vi "ep_Get Significance.vi"(0 "spectra points in window":T4(array[cluster]), 1 "pole pairs":i32, 2 "fundamental frequency [Hz]":dbl, 5 "peaks information":T3(array[cluster]), 7 "enough points for peak search?":bool[](array[boolean]), 9 "number of peaks":i32[](array[numeric]), 11 "error in (no error)":errorcluster, 12 "minimum max-magnitude":dbl, 13 "range of speed":T1) -> (4 "top3 speed data":cluster{"speed [RPM]":dbl, "slip":dbl}[](array[cluster]), 6 "top3 significance":dbl[](array[numeric]), 8 "top3 harmonic for speed calculation":T2[](array[typedef]), 15 "error out":errorcluster)   [LabVIEW 2014, in "NI_EP_Motor Monitoring.lvlib"]
uses:
  <vilib>/addons/Electrical Power/Motor Monitoring/NI_EP_Motor Monitoring.lvlib
  <vilib>/addons/Electrical Power/Motor Monitoring/subVIs/ep_Harmonic for Speed Calculation.ctl
  <vilib>/Analysis/baseanly.llb/Mean (DBL).vi
  <vilib>/Analysis/NI_AALBase.lvlib
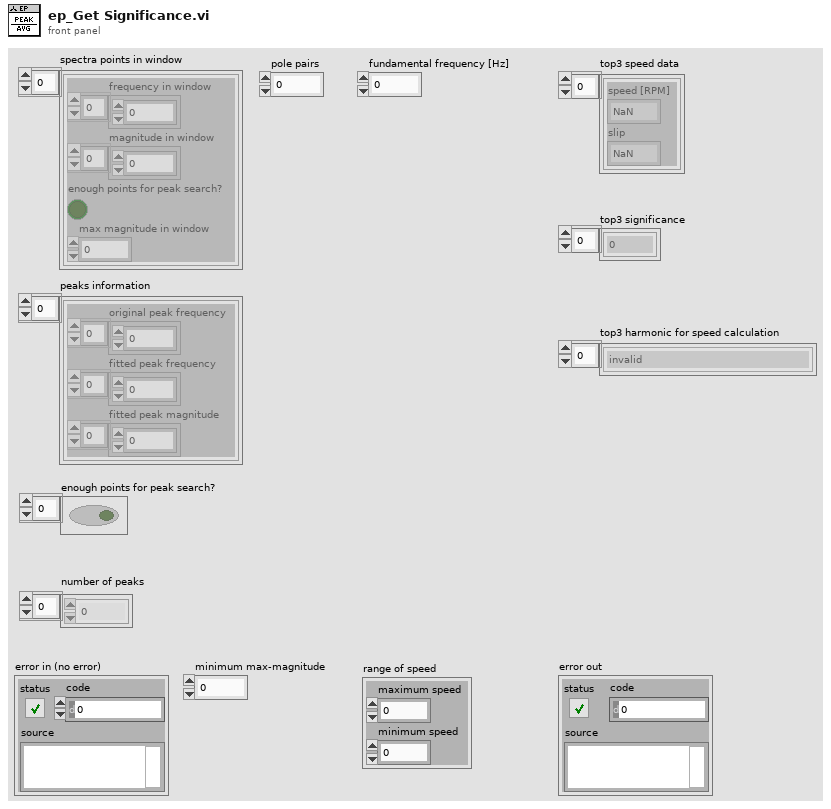
[diagram p1: front panel]
types:
  T1 = cluster{"maximum speed":dbl, "minimum speed":dbl}
  T2 = typedef "NI_EP_Motor Monitoring.lvlib/ep_Harmonic for Speed Calculation.ctl" = enum16{"invalid", "fr", "2fs-2fr", "2fs-fr", "2fr"}
  T3 = cluster{"original peak frequency":dbl[], "fitted peak frequency":dbl[], "fitted peak magnitude":dbl[]}[]
  T4 = cluster{"frequency in window":dbl[], "magnitude in window":dbl[], "enough points for peak search?":bool, "max magnitude in window":dbl}[]
  T5 = typedef "NI_EP_Motor Monitoring.lvlib/ep_Case for Speed Calculation.ctl" = enum16{"no available harmonic for speed calculation", "use the harmonic with highest magnitude", "use the harmonic with highest significance"}
  T6 = cluster{"frequency in window":dbl[], "magnitude in window":dbl[], "enough points for peak search?":bool, "max magnitude in window":dbl}
  T7 = cluster{"maximum frequency [Hz]":dbl, "slip error allowance":dbl, "minimum points for peak search":dbl, "accuracy of fs":dbl, "difference?":bool, " fs harmonics order":i32, "fs forbidden range":dbl, "p3:p1 valid significance ratio":dbl, "ratio for significance weighting":dbl, "significance weighting":dbl}
  T8 = cluster{"original peak frequency":dbl[], "fitted peak frequency":dbl[], "fitted peak magnitude":dbl[]}
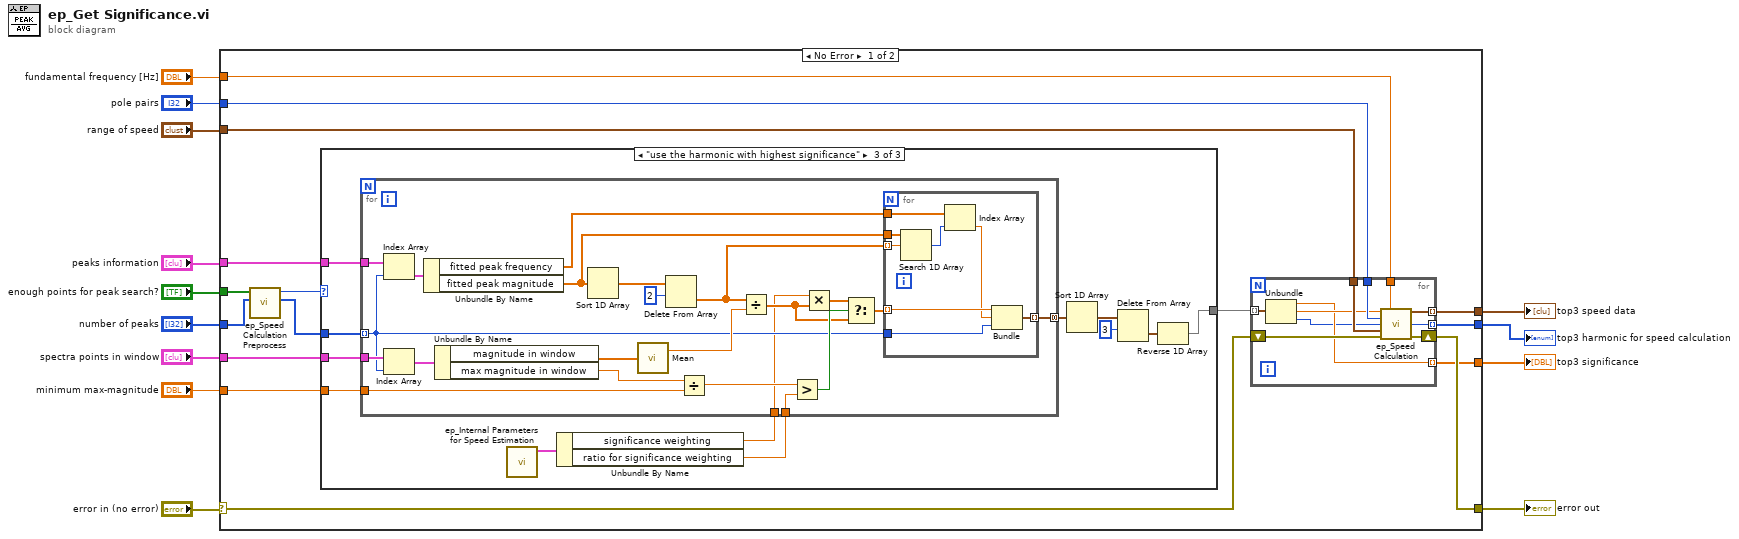
[diagram p0: block diagram]
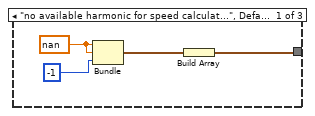
[diagram p2: hidden frame]
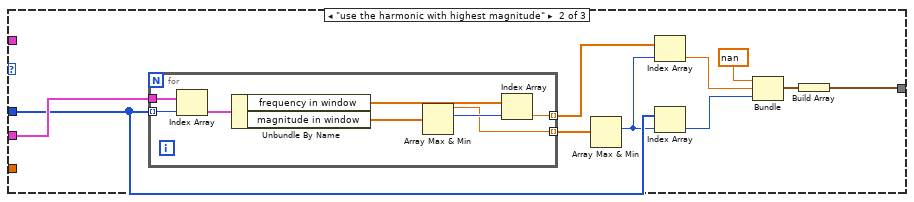
[diagram p3: hidden frame]
diagram:
  n1 = case shown="No Error" "error in (no error)" {
    selector: "error in (no error)" -> [w26 w105]
    tunnel: [w25 w105] -> w12
    tunnel: "peaks information" -> [w29 _]
    tunnel: "spectra points in window" -> [w27 _]
    tunnel: [w28 _] -> w9
    tunnel: [w24 _] -> w8
    tunnel: "fundamental frequency [Hz]" -> [w23 _]
    tunnel: "pole pairs" -> [w22 _]
    tunnel: "range of speed" -> [w21 _]
    tunnel: [w19 _] -> w4
    tunnel: "minimum max-magnitude" -> [w18 _]
    tunnel: "enough points for peak search?" -> [w15 _]
    tunnel: "number of peaks" -> [w14 _]
    frame No Error {
      n2 = call <vilib>:"ep_Speed Calculation Preprocess.vi"("number of peaks"=w14, "enough points for peak search?"=w15) -> ("harmonic for comparison"=w16:i32[], "case for speed calculation"=w17:T5)  [unwired: 8 in]
      n3 = case shown="\"use the harmonic with highest significance\"" w17 {
        tunnel: w29 -> [_ _ w74]
        tunnel: w27 -> [_ w54 w72]
        tunnel: w16 -> [_ w52 w73]
        tunnel: [w41 w48 w67] -> w20
        tunnel: w18 -> [_ _ w65]
        frame "no available harmonic for speed calculation", Default {
          w44 = nan
          n4 = Bundle(w44, w44, -1) -> (w42:cluster{dbl, dbl, i32})  [unwired: 1 in]
          n5 = Build Array(w42) -> (w41:cluster{dbl, dbl, i32}[])
        }
        frame "use the harmonic with highest magnitude" {
          n6 = for {
            tunnel: w52 -> [w61] mode=indexing
            tunnel: w54 -> [w62]
            tunnel: [w56] -> w53 mode=indexing
            tunnel: [w55] -> w51 mode=indexing
            n7 = Index Array(array=w62, index=w61) -> (element=w60:T6)
            n8 = Unbundle By Name(w60) -> ("frequency in window"=w58:dbl[], "magnitude in window"=w59:dbl[])
            n9 = Array Max & Min(array=w59) -> (max value=w56:dbl, max index (indices)=w57:i32)  [unwired: 2 out]
            n10 = Index Array(array=w58, index=w57) -> (element=w55:dbl)
          }
          n11 = Array Max & Min(array=w53) -> (max index (indices)=w50:i32)  [unwired: 3 out]
          n12 = Index Array(array=w51, index=w50) -> (element=w46:dbl)
          n13 = Index Array(array=w52, index=w50) -> (element=w45:i32)
          n14 = Bundle(nan, "frequency points"=w46, w45) -> (w47:cluster{dbl, "frequency points":dbl, i32})  [unwired: 1 in]
          n15 = Build Array(w47) -> (w48:cluster{dbl, "frequency points":dbl, i32}[])
        }
        frame "use the harmonic with highest significance" {
          n16 = call <vilib>:"ep_Internal Parameters for Speed Estimation.vi"() -> ("internal parameters for speed estimation"=w66:T7)  [unwired: 11 in]
          n17 = Unbundle By Name(w66) -> ("significance weighting"=w63:dbl, "ratio for significance weighting"=w64:dbl)
          n18 = for {
            tunnel: w74 -> [w96]
            tunnel: w73 -> [w83] mode=indexing
            tunnel: w72 -> [w93]
            tunnel: [w82] -> w71 mode=concatenating
            tunnel: w65 -> [w77]
            tunnel: w64 -> [w76]
            tunnel: w63 -> [w75]
            n19 = Index Array(array=w96, index=w83) -> (element=w94:T8)
            n20 = Index Array(array=w93, index=w83) -> (element=w88:T6)
            n21 = Unbundle By Name(w94) -> ("fitted peak frequency"=w95:dbl[], "fitted peak magnitude"=w92:dbl[])
            n22 = Unbundle By Name(w88) -> ("magnitude in window"=w87:dbl[], "max magnitude in window"=w78:dbl)
            n23 = Sort 1D Array(array=w92) -> (sorted array=w81:dbl[])
            n24 = call-poly <vilib>:"Mean.vi"("X"=w87) -> ("mean"=w89:dbl)  [unwired: 1 out]
            n25 = Delete From Array(array=w81, length=2 ("index")) -> (deleted portion=w79:dbl[])  [unwired: 1 in, 1 out]
            n26 = Divide(x=w78, y=w77) -> (x/y=w91:dbl)
            n27 = Divide(x=w79, y=w89) -> (x/y=w85:dbl[])
            n28 = Greater?(x=w91, y=w76) -> (0:w90:bool)
            n29 = Multiply(x=w75, y=w85) -> (x*y=w86:dbl[])
            n30 = Select(t=w86, s=w90, f=w85) -> (s? t:f=w84:dbl[])
            n31 = for {
              tunnel: w95 -> [w103]
              tunnel: w79 -> [w104] mode=indexing
              tunnel: w92 -> [w102]
              tunnel: w84 -> [w100] mode=indexing
              tunnel: w83 -> [w99]
              tunnel: [w98] -> w82 mode=indexing
              n32 = Search 1D Array(1D array=w102, element=w104) -> (index of element=w101:i32)  [unwired: 1 in]
              n33 = Index Array(array=w103, index=w101) -> (element=w97:dbl)
              n34 = Bundle(w100, w97, w99) -> (w98:cluster{dbl, dbl, i32})  [unwired: 1 in]
            }
          }
          n35 = Sort 1D Array(array=w71) -> (sorted array=w69:cluster{dbl, dbl, i32}[])
          n36 = Delete From Array(array=w69, length=3 ("index")) -> (deleted portion=w68:cluster{dbl, dbl, i32}[])  [unwired: 1 in, 1 out]
          n37 = Reverse 1D Array(array=w68) -> (reversed array=w67:cluster{dbl, dbl, i32}[])
        }
      }
      n38 = for {
        tunnel: [w30] -> w28 mode=indexing
        shift-right: [w39] -> w25
        shift-left: w26 -> [w40]
        tunnel: [w38] -> w24 mode=indexing
        tunnel: w23 -> [w37]
        tunnel: w22 -> [w36]
        tunnel: w21 -> [w35]
        tunnel: w20 -> [w34] mode=indexing
        tunnel: [w32] -> w19 mode=indexing
        n39 = Unbundle(w34) -> (w32:dbl, "frequency points"=w33:dbl, w31:i32)
        n40 = call <vilib>:"ep_Speed Calculation.vi"("harmonic frequency"=w33, "fundamental frequency [Hz]"=w37, "pole pairs"=w36, "harmonic for speed calculation"=w31, "range of speed"=w35, "error in (no error)"=w40) -> ("speed data"=w38:cluster{"speed [RPM]":dbl, "slip":dbl}, "harmonic for speed calculation"=w30:T2, "error out"=w39:errorcluster)  [unwired: 7 in]
      }
    }
    frame Error {
    }
  }
  "error out" <- w12
  "top3 harmonic for speed calculation" <- w9
  "top3 significance" <- w4
  "top3 speed data" <- w8
